vi "AfterLoad.vi"(8 "error in (no error)":errorcluster, 11 "SettingsFileIQpid in":refnum<class "SettingsFileIQpid.lvclass">) -> (0 "error out":errorcluster, 3 "SettingsFileIQpid out":refnum<class "SettingsFileIQpid.lvclass">)   [LabVIEW 2018, in "SettingsFileIQpid.lvclass"]
uses:
  SettingsFileIQpid.lvclass
  SettingsFileIQpid.lvclass/SettingsFileIQpid.ctl
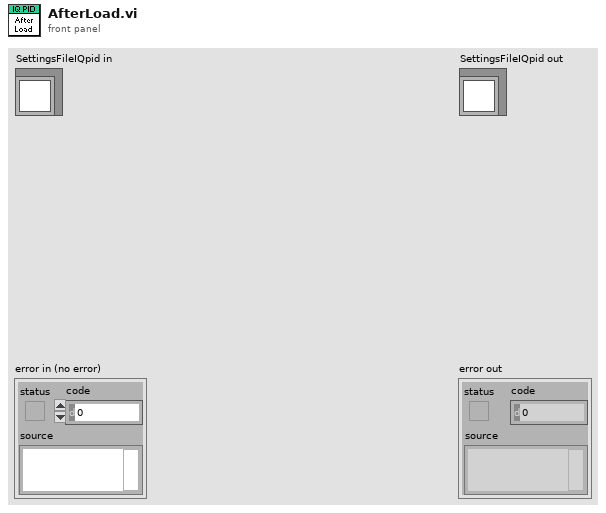
[diagram p1: front panel]
types:
  T1 = typedef "All FP controls.ctl" = cluster{"Adaptive FF enabled":refnum<vi>, "LP filter cutoff fequency [MHz]":refnum<vi>, "Adaptation factor [0-1]":refnum<vi>, "Samples to skip":refnum<vi>, "ch1 DC offset":refnum<vi>, "ch0 DC offset":refnum<vi>, "ch1 DC offset 2":refnum<vi>, "ch0 DC offset 2":refnum<vi>, "ch3 DC offset":refnum<vi>, "ch2 DC offset":refnum<vi>, "Feedback Q":refnum<vi>, "Ki*T Q":refnum<vi>, "Kd/T  Q":refnum<vi>, "Kp Q":refnum<vi>, "Acquire samples":refnum<vi>, "Trigger delay":refnum<vi>, "Feedback delay":refnum<vi>, "Kp AM":refnum<vi>, "Kd/T AM":refnum<vi>, "Ki*T AM":refnum<vi>, "Feedback I":refnum<vi>, "#bins":refnum<vi>, "Window":refnum<vi>, "Unit":refnum<vi>, "Input delay 5761":refnum<vi>, "Input delay 5785":refnum<vi>, "S":refnum<vi>, "K1":refnum<vi>, "Q1":refnum<vi>, "R1":refnum<vi>, "w12":refnum<vi>, "Cavity model":refnum<vi>, "w1":refnum<vi>, "Mode":refnum<vi>, "Trigger":refnum<vi>, "Output mixer fequency [MHz]":refnum<vi>, "Output delay":refnum<vi>, "Mixer freq [MHz]":refnum<vi>, "Triggered":refnum<vi>, "Continuous":refnum<vi>, "Output scale":refnum<vi>, "Host scale":refnum<vi>, "Input scale":refnum<vi>, "IIR filter cutoff fequency [MHz]":refnum<vi>, "Host scale 5761":refnum<vi>, "Virtual cavity":refnum<vi>, "Input scale 5761":refnum<vi>, "Tranfer speed":refnum<vi>, "Count to skip 5782":refnum<vi>, "Count to skip 5761":refnum<vi>, "K2":refnum<vi>, "w2":refnum<vi>, "K3":refnum<vi>, "Q3":refnum<vi>, "Q2":refnum<vi>, "w3":refnum<vi>, "w0":refnum<vi>, "Piezo":refnum<vi>}
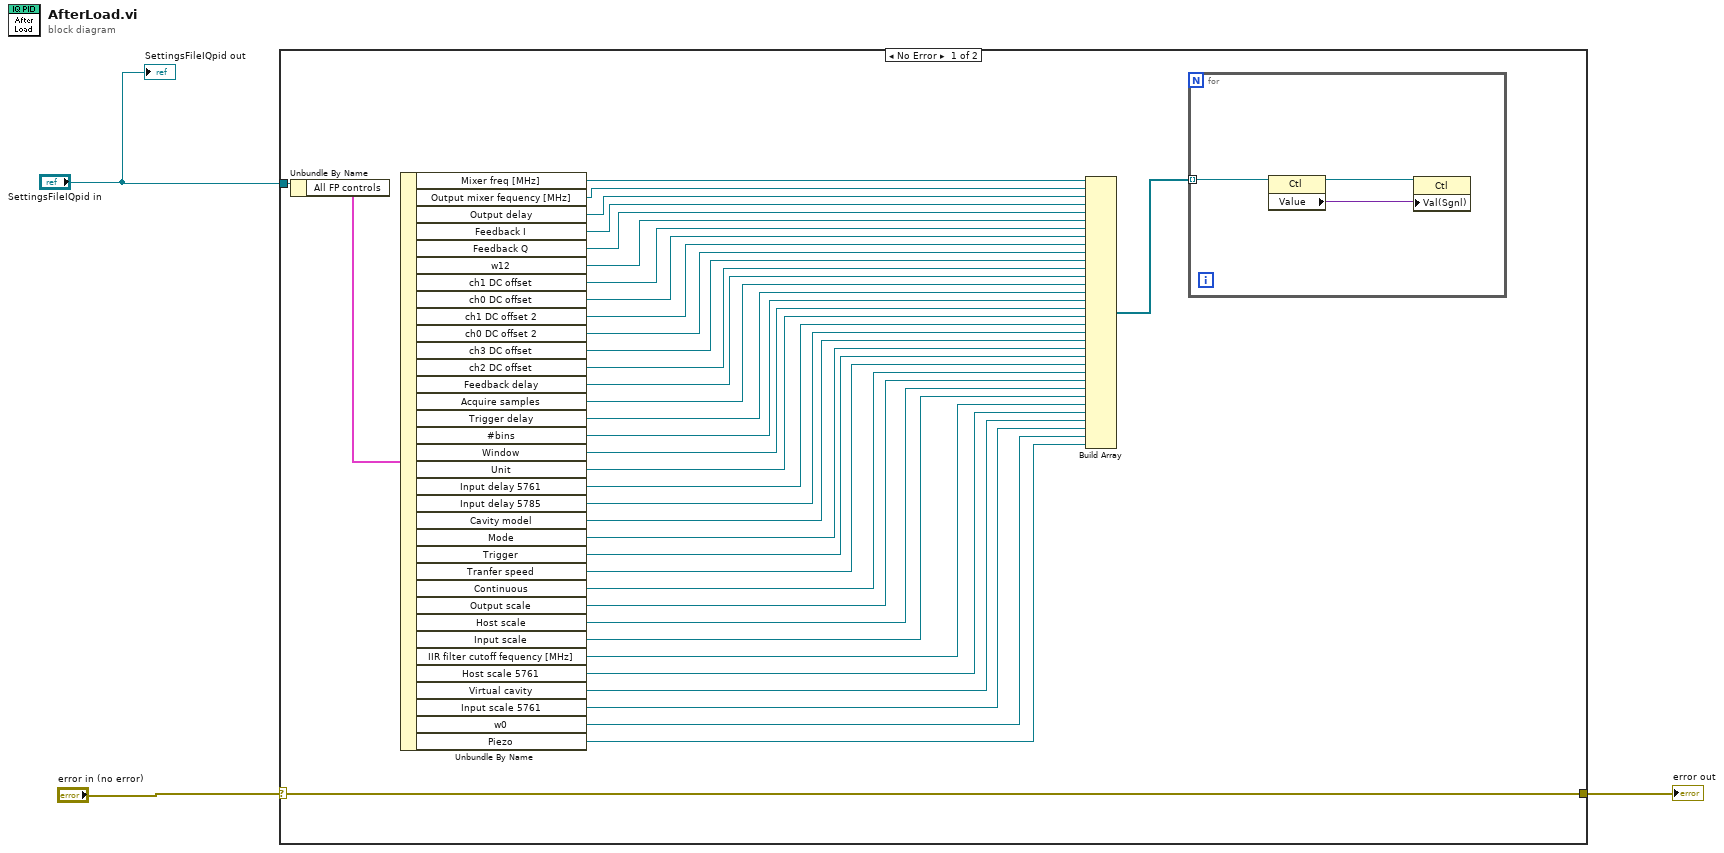
[diagram p0: block diagram]
diagram:
  n1 = case shown="No Error" "error in (no error)" {
    selector: "error in (no error)" -> [w13 w45]
    tunnel: "SettingsFileIQpid in" -> [w39 _]
    tunnel: [w13 w45] -> w1
    frame No Error {
      n2 = Unbundle By Name(w39) -> ("All FP controls"=w41:T1)
      n3 = Unbundle By Name(w41) -> ("Mixer freq [MHz]"=w40:refnum<vi>, "Output mixer fequency [MHz]"=w38:refnum<vi>, "Output delay"=w37:refnum<vi>, "Feedback I"=w36:refnum<vi>, "Feedback Q"=w35:refnum<vi>, "w12"=w34:refnum<vi>, "ch1 DC offset"=w33:refnum<vi>, "ch0 DC offset"=w32:refnum<vi>, "ch1 DC offset 2"=w31:refnum<vi>, "ch0 DC offset 2"=w30:refnum<vi>, "ch3 DC offset"=w29:refnum<vi>, "ch2 DC offset"=w28:refnum<vi>, "Feedback delay"=w27:refnum<vi>, "Acquire samples"=w26:refnum<vi>, "Trigger delay"=w24:refnum<vi>, "#bins"=w23:refnum<vi>, "Window"=w22:refnum<vi>, "Unit"=w21:refnum<vi>, "Input delay 5761"=w20:refnum<vi>, "Input delay 5785"=w19:refnum<vi>, "Cavity model"=w18:refnum<vi>, "Mode"=w17:refnum<vi>, "Trigger"=w16:refnum<vi>, "Tranfer speed"=w15:refnum<vi>, "Continuous"=w14:refnum<vi>, "Output scale"=w12:refnum<vi>, "Host scale"=w11:refnum<vi>, "Input scale"=w9:refnum<vi>, "IIR filter cutoff fequency [MHz]"=w10:refnum<vi>, "Host scale 5761"=w8:refnum<vi>, "Virtual cavity"=w7:refnum<vi>, "Input scale 5761"=w6:refnum<vi>, "w0"=w5:refnum<vi>, "Piezo"=w4:refnum<vi>)
      n4 = Build Array(w40, w38, w37, w36, w35, w34, w33, w32, w31, w30, w29, w28, w27, w26, w24, w23, w22, w21, w20, w19, w18, w17, w16, w15, w14, w12, w11, w9, w10, w8, w7, w6, w5, w4) -> (w25:refnum<vi>[])
      n5 = for {
        tunnel: w25 -> [w44] mode=indexing
        n6 = property class="Ctl"(reference=w44) -> (reference out=w42:refnum<vi>, "Value"=w43:variant)  [unwired: 1 in, 1 out]
        n7 = property class="Ctl"(reference=w42, "Val(Sgnl)"=w43) -> ()  [unwired: 1 in, 2 out]
      }
    }
    frame Error {
    }
  }
  "error out" <- w1
  "SettingsFileIQpid out" <- "SettingsFileIQpid in"
